vi "Solve1.vi"(8 "Error In":errorcluster, 11 "object in":refnum<class "2021_1.lvclass">) -> (0 "Error Out":errorcluster, 2 "Result":u64, 3 "object out":refnum<class "2021_1.lvclass">)   [LabVIEW 2020, in "2021_1.lvclass"]
uses:
  2021_1.lvclass
  2021_1.lvclass/2021_1.ctl
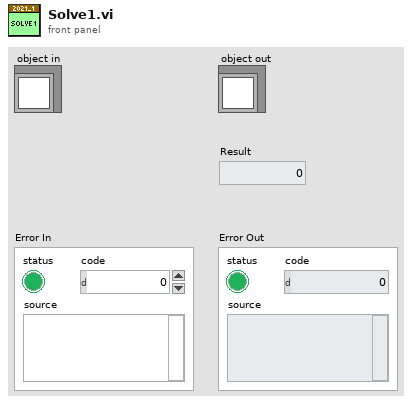
[diagram p1: front panel]
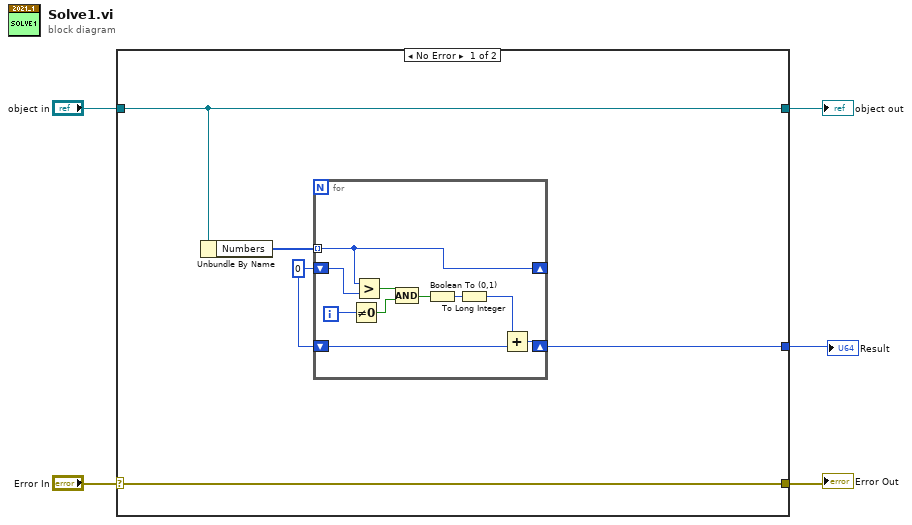
[diagram p0: block diagram]
diagram:
  n1 = case shown="No Error" "Error In" {
    selector: "Error In" -> [w10 w22]
    tunnel: [w10 w22] -> w4
    tunnel: [w9 w21] -> w2
    tunnel: "object in" -> [w9 w21]
    tunnel: [w6 _] -> w1
    frame No Error {
      w7 = 0
      n2 = Unbundle By Name(w9) -> ("Numbers"=w8:i32[])
      n3 = for {
        tunnel: w8 -> [w20] mode=indexing
        shift-right: [w20] -> _
        shift-left: w7 -> [w19]
        shift-right: [w12] -> w6
        shift-left: w7 -> [w13]
        i -> [w16]
        n4 = Not Equal To 0?(x=w16) -> (x != 0?=w17:bool)
        n5 = Greater?(x=w20, y=w19) -> (0:w18:bool)
        n6 = Compound Arithmetic op=AND(w18, w17) -> (w15:bool)
        n7 = Boolean To (0,1)(Boolean=w15) -> (0, 1=w14:i16)
        n8 = To Long Integer(number=w14) -> (32bit integer=w11:i32)
        n9 = Add(x=w11, y=w13) -> (x+y=w12:i32)
      }
    }
    frame Error {
    }
  }
  "Error Out" <- w4
  "object out" <- w2
  "Result" <- w1
